vi "SV Global.vi"() -> ()   [LabVIEW 2021]
panel:
  in  "CD Version":string="2.0.1"
  in  "Supported File Formats":string="*.ini;*.txt;*.json"
  in  "Version":string="NI VeriStand 2021"
  in  "SV Update Rate":string
  in  "Target":string="Target"
  in  "Status":string="Status"
  in  "Shared Variable Name":string="Shared Variable Name"
  in  "Shared Variable URL":string="Shared Variable URL"
  in  "Channel Type":string="Channel Type"
  in  "Write":string="Write"
  in  "Read":string="Read"
  in  "Error Code":string="Error Code"
  in  "Timeout":string="Timeout"
  in  "Localhost IP Address":string="localhost"
  in  "PSP URL":string="ni.var.psp://"
  # "Import Export"
  # "Shared Variable Info"
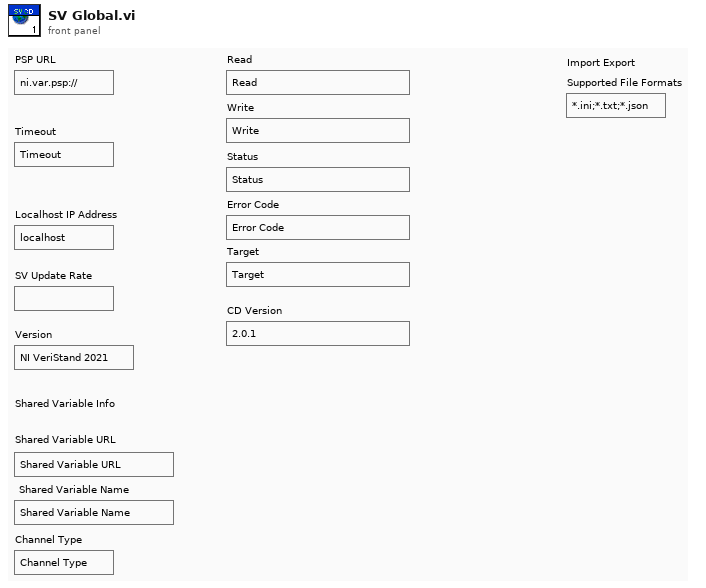
[diagram p1: front panel]
diagram:
